vi "Invert.vi"(8 "error in":errorcluster, 11 "Orient3d in":refnum<class "Orient3d.lvclass">) -> (0 "error out":errorcluster, 3 "Orient3d out":refnum<class "Orient3d.lvclass">)   [LabVIEW 2024, in "Orient3d.lvclass"]
uses:
  Orient3d.lvclass
  <vilib>/Analysis/7linalg.llb/Real Transpose Matrix.vi
  <vilib>/Analysis/NI_AALPro.lvlib
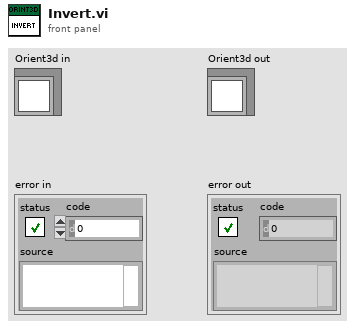
[diagram p1: front panel]
types:
  T1 = typedef "NI_Matrix.lvlib/RealMatrix.ctl" = dbl[][]
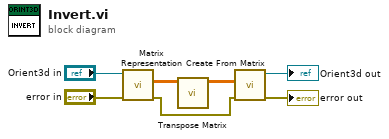
[diagram p0: block diagram]
diagram:
  n1 = call "Matrix Representation.vi"("error in"="error in", "Orient3d in"="Orient3d in") -> ("error out"=w3:errorcluster, "Rotation Matrix"=w5:T1)  [unwired: 7 in, 1 out]
  n2 = call-poly <vilib>:"Transpose Matrix.vi"("Input Matrix"=w5) -> ("Matrix Transpose"=w4:T1)  [unwired: 9 in, 1 out]
  n3 = call "Create From Matrix.vi"("error in"=w3, "Rotation Matrix"=w4) -> ("error out"=→"error out":errorcluster, "Orient3d out"=→"Orient3d out":refnum<class "Orient3d.lvclass">)  [unwired: 8 in]
